vi "Move_Files_Gain.vi"(6 "Folder name":string, 7 "Run":string, 8 "PMTs":string[](array[string]), 9 "Channel":string[](array[string]), 10 "Folder Containing Bash Script":string="Wavedump_Bash_Script_Test_", 11 "Name of Folder to\nCopy PMT File to":string) -> ()   [LabVIEW 2019]
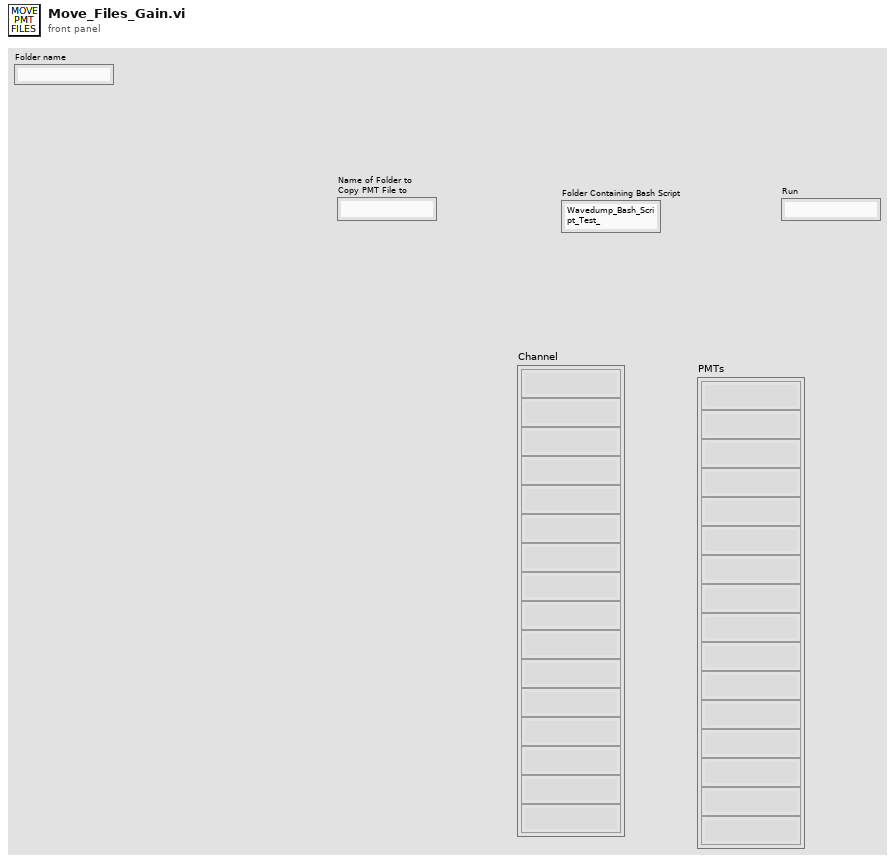
[diagram p1: front panel]
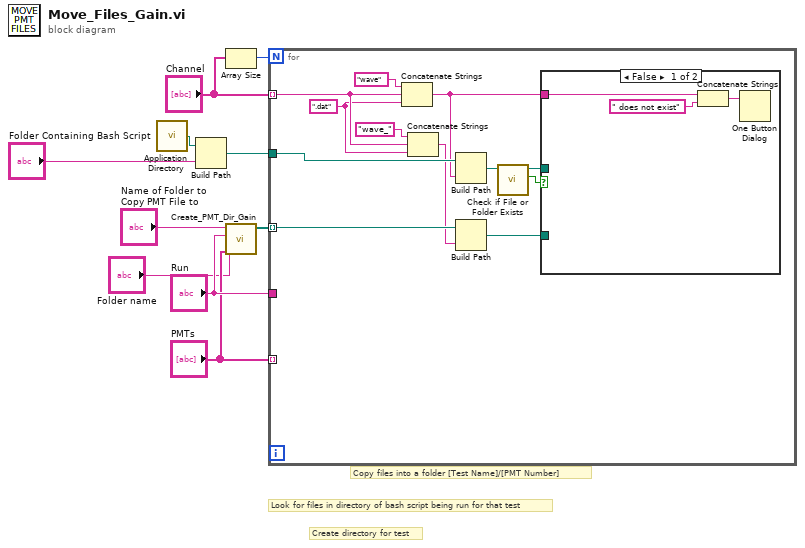
[diagram p0: block diagram]
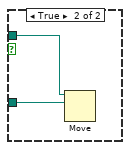
[diagram p2: hidden frame]
diagram:
  # "Create directory for test"
  # "Look for files in directory of bash script being run for that test"
  # "Copy files into a folder [Test Name]/[PMT Number]"
  n1 = call <vilib>:"Application Directory.vi"() -> ("Application Directory"=w10:path)
  n2 = Build Path(base path=w10, name or relative path="Folder Containing Bash Script") -> (appended path=w6:path)
  n3 = Array Size(array="Channel") -> (size(s)=w8:i32)
  n4 = call "Create_PMT_Dir_Gain.vi"("Test"="Name of Folder to\nCopy PMT File to", "Run"="Run", "Folder name"="Folder name", "PMTs"="PMTs") -> ("Paths"=w5:path[])  [unwired: 6 in]
  n5 = for {
    N: w8 -> [_]
    tunnel: w5 -> [w20] mode=indexing
    tunnel: w6 -> [w21]
    tunnel: "Channel" -> [w18] mode=indexing
    tunnel: "Run" -> [_]
    tunnel: "PMTs" -> [_] mode=indexing
    w17 = ".dat" ("string")
    n6 = Concatenate Strings("wave" ("string"), w18, w17) -> (w11:string)
    n7 = Concatenate Strings("wave_" ("string"), w18, w17) -> (w19:string)
    n8 = Build Path(base path=w21, name or relative path=w11) -> (appended path=w15:path)
    n9 = Build Path(base path=w20, name or relative path=w19) -> (appended path=w13:path)
    n10 = call <vilib>:"Check if File or Folder Exists.vi"("path"=w15) -> ("file or folder exists?"=w14:bool, "dup path"=w12:path)  [unwired: 8 in, 1 out]
    n11 = case shown="False" w14 {
      tunnel: w13 -> [_ w27]
      tunnel: w12 -> [_ w26]
      tunnel: w11 -> [w24 _]
      frame False {
        n12 = Concatenate Strings(w24, " does not exist" ("string")) -> (w25:string)
        n13 = One Button Dialog(message=w25) -> ()  [unwired: 1 in, 1 out]
      }
      frame True {
        n14 = Move(source path=w26, 10:w27) -> ()  [unwired: 3 in, 3 out]
      }
    }
  }
